vi "Test Copy Image to Pixmap No Mask Greyscale.vi"(8 "error in (no error)":errorcluster, 11 "Test Case In":refnum<class "Image.lvclass">) -> (0 "error out":errorcluster, 3 "Test Case Out":refnum<class "Image.lvclass">)   [LabVIEW 2020, in "g_ar_toolkit.test.lvlib" / "Image.lvclass"]
uses:
  Image.lvclass
  C:/Program Files (x86)/National Instruments/LabVIEW 2020/vi.lib/Astemes/LUnit/Test Case.lvclass
  g_ar_toolkit.common/Image Size (Integer).ctl
  <vilib>/Astemes/LUnit/Test Case.lvclass/Test Case.ctl
  g_ar_toolkit.image/Copy Image to Pixmap Greyscale.vi
  4993e8ee-a06a-463a-9684-69129f64d5ce.vi
  g_ar_toolkit.image/New Image.vi
  g_ar_toolkit.image/New Image (Greyscale).vi
  g_ar_toolkit.image/Copy Array to Image.vi
  g_ar_toolkit.image/Copy Array to Image (Greyscale).vi
  g_ar_toolkit.image/Copy Image to Pixmap Greyscale.vi/5c639587-cf36-4d54-93d9-e654c7c24c6e.vi
  <vilib>/Astemes/LUnit/Append Pass Result.vi
  <vilib>/Astemes/LUnit/Append Fail Result.vi
  <vilib>/Astemes/LUnit/Describe Comparison.vi
  4993e8ee-a06a-463a-9684-69129f64d5ce.vi/9c5d11cd-9439-4240-a1ee-d9baace9c924.vi
  g_ar_toolkit.image/New Image (Greyscale).vi/6598b9e0-8a08-46f5-91fd-ca1b87217137.vi
  <vilib>/Astemes/LUnit/Run In UI.vi
  <vilib>/Utility/error.llb/Clear Errors.vi
  g_ar_toolkit.common/Module Path.vi
  <vilib>/Utility/error.llb/Error Cluster From Error Code.vi
  <vilib>/picture/pixmap.llb/Flatten Pixmap.vi
  <vilib>/Astemes/LUnit/Describe Variant.vi
  Image.lvclass/Image.ctl
  g_ar_toolkit.common/g_ar_toolkit.common.lvlib
  g_ar_toolkit.image/g_ar_toolkit.image.lvlib
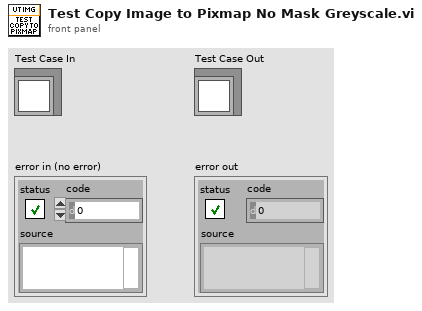
[diagram p1: front panel]
types:
  T1 = typedef "g_ar_toolkit.common.lvlib/Image Size (Integer).ctl" = cluster{"Width":u16, "Height":u16}
  T2 = typedef "g_ar_toolkit.image.lvlib/Greyscale Image.ctl" = refnum<data-value>
  T3 = typedef "imagedata.ctl" = cluster{"image type":i32, "image depth":i32, "image":u8[], "mask":u8[], "colors":u32[], "Rectangle":cluster{"left":i16, "top":i16, "right":i16, "bottom":i16}}
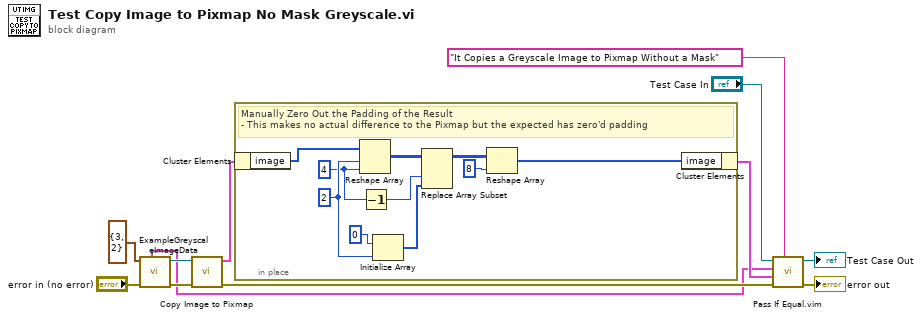
[diagram p0: block diagram]
diagram:
  n1 = call "ExampleGreyscaleImageData.vi"("error in (no error)"="error in (no error)", "Image Size"=T1 {"Width"=3, "Height"=2} ("Preallocated Image Size (Default - 0,0)")) -> ("error out"=w8:errorcluster, "Greyscale Destination Image"=w5:T2, "Greyscale Pixmap Data"=w1:T3)  [unwired: 6 in, 1 out]
  n2 = call-poly "Copy Image to Pixmap.vi"("error in (no error)"=w8, "Greyscale Image Source"=w5) -> ("error out"=w4:errorcluster, "Pixmap Image Data"=w3:T3)  [unwired: 8 in]
  n3 = in-place {
    w16 = 4 ("dimension size")
    w20 = 2 ("dimension size")
    # "Manually Zero Out the Padding of the Result\n- This makes no actual difference to the Pixmap but the expected has zero'd padding"
    n4 = in-place-cluster #1(w3) -> ("image"=w22:u8[])
    n5 = Reshape Array(w22, w20, w16) -> (w21:u8[][])
    n6 = Decrement(x=w16) -> (x-1=w17:i32)
    n7 = Initialize Array(u8 0 ("element"), w20) -> (w18:u8[])
    n8 = Replace Array Subset(array=w21, new element=w18, index (col)=w17) -> (w15:u8[][])  [unwired: 1 in]
    n9 = Reshape Array(w15, 8 ("dimension size")) -> (w14:u8[])
    n10 = in-place-cluster #1("image"=w14) -> (w2:T3)
  }
  n11 = call "Pass If Equal.vim"("Description"="It Copies a Greyscale Image to Pixmap Without a Mask", "error in (no error)"=w4, "Actual"=w2, "Expected"=w1, "LUnit Test Case In"="Test Case In") -> ("error out"=→"error out":errorcluster, "LUnit Test Case Out"=→"Test Case Out":refnum<class "Image.lvclass">)  [unwired: 5 in]
